vi "te_writeVal.vi"(0 "VISA In":refnum<visa-resource-name>, 5 "Hex Address":string="00", 7 "Command":string="01", 9 "Data":i32, 11 "Error In":errorcluster) -> (4 "VISA Out":refnum<visa-resource-name>, 6 "Response Dec":dbl, 8 "Response":dbl, 15 "error out":errorcluster)   [LabVIEW 2018]
doc: "The Basic Serial Read and Write example performs a Serial Port Read, a Serial Port Write, or a combination of these actions. The user selects the actions (read or write) on the front panel. If both are selected, the VI will write the data first, read data, and then close the VISA session that is opened to the port. This VI will wait until the specified number of bytes is received at the port. Only the number of bytes specified will be read.\n\nINSTRUCTIONS:\n1) Select the serial resource and configuration parameters (baud rate, data bits, parity, stop bits, flow control).\n2) Select the operations to be performed. \n3) Connect the serial port to your device. If no device is available, perform a loopback test by doing one of the following. Short pins 2 and 3 on a RS-232 cable or short pin 4 to pin 8 and pin 5 to pin 9 on a RS-485/422 cable. \n4) Run the VI to see the data read. (The \"read string\" will match the \"string to write\" if a loopback test was performed.)\n\nNote: The parameters set for the serial port must match the parameters of the connected instrument or device. In this example, the bytes to read parameter specifies the number of bytes that the serial port reads. If there were more bytes at the port than the number specified in bytes to read, those bytes would not be read. Also, if you specify to read more bytes than the number of bytes actually read, you might receive a timeout error message.\n\nOn the block diagram, the Configure Serial Port VI sets the configuration parameters. The front panel displays the controls used to configure the basic parameters, such as baud rate, data bits, and parity. Constants configure the other parameters the user probably does not need set. After the VISA Configure Serial Port VI opens the VISA session and configures the port, the VI passes the VISA resource name to other VIs that perform operations on that VISA resource. The VISA Write function sends a command to the serial device and the VISA Read function returns data based on the command. The VISA Close function then closes the reference to the serial device. It is important to close the reference; otherwise communication through with that port through protocols other than VISA might not be possible."
panel:
  out "Response Hex":string
  out "Checksum":string
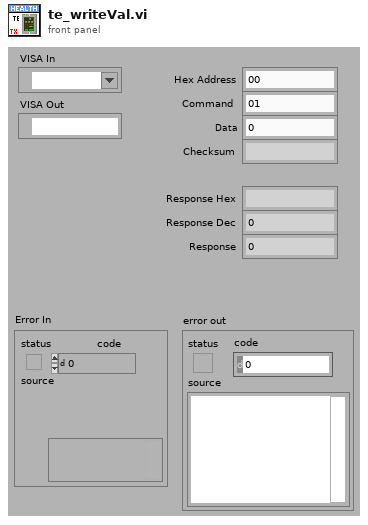
[diagram p1: front panel]
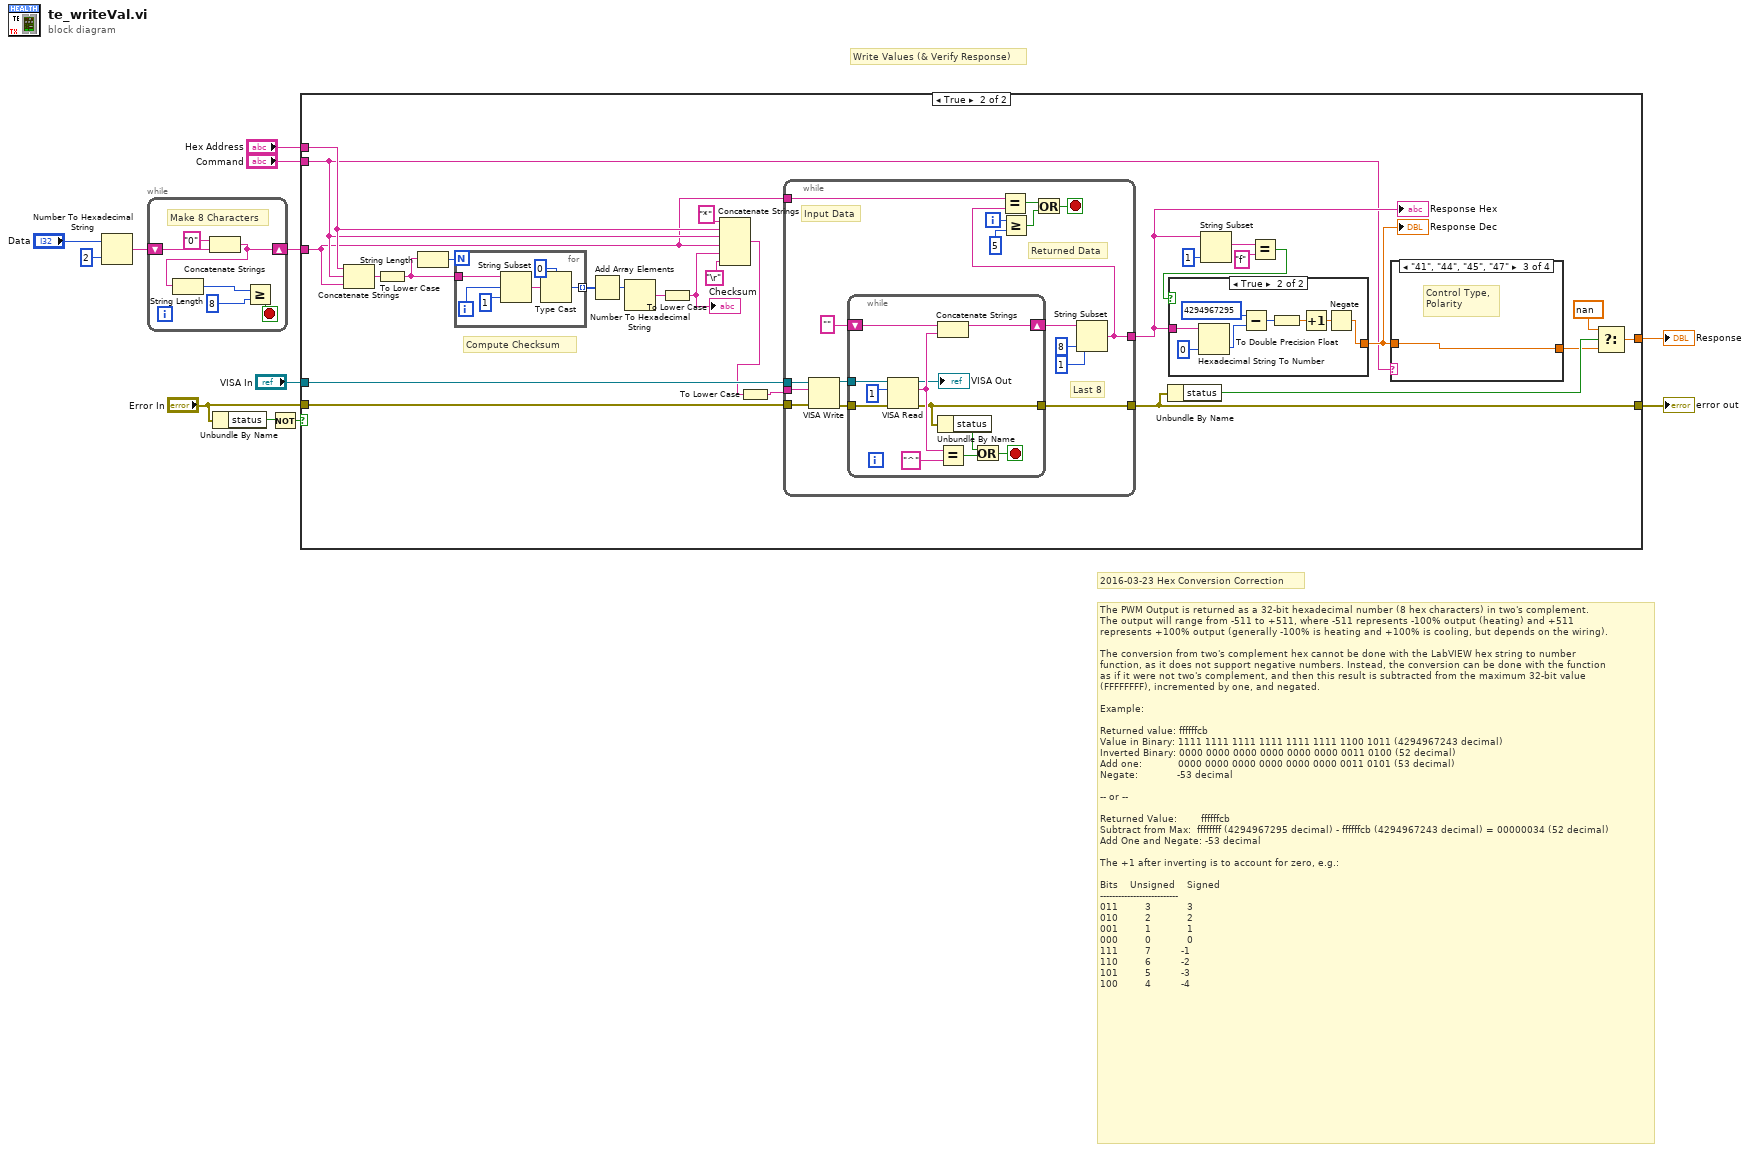
[diagram p0: block diagram]
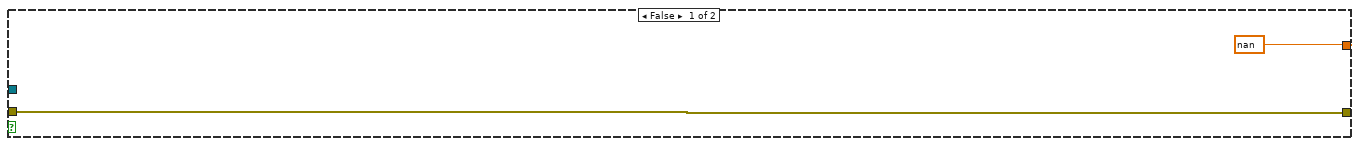
[diagram p2: hidden frame]
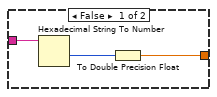
[diagram p3: hidden frame]
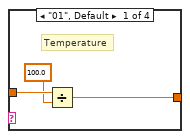
[diagram p4: hidden frame]
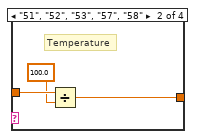
[diagram p5: hidden frame]
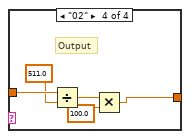
[diagram p6: hidden frame]
diagram:
  # "Write Values (& Verify Response)"
  # "2016-03-23 Hex Conversion Correction"
  # "The PWM Output is returned as a 32-bit hexadecimal number (8 hex characters) in two's complement.\nThe output will range from -511 to +511, where -511 represents -100% output (heating) and +511\nrepresents +100% output (generally -100% is heating and +100% is cooling, but depends on the wiring).\n\nThe conversion from two's complement hex cannot be done with the LabVIEW hex string to number\nfunction, as it does not support negative numbers. Instead, the conversion can be done with the function\nas if it were not two's complement, and then this result is subtracted from the maximum 32-bit value\n(FFFFFFFF), incremented by one, and negated.\n\nExample:\n\nReturned value: ffffffcb\nValue in Binary: 1111 1111 1111 1111 1111 1111 1100 1011 (4294967243 decimal)\nInverted Binary: 0000 0000 0000 0000 0000 0000 0011 0100 (52 decimal)\nAdd one:            0000 0000 0000 0000 0000 0000 0011 0101 (53 decimal)\nNegate:             -53 decimal\n\n-- or --\n\nReturned Value:        ffffffcb\nSubtract from Max:  ffffffff (4294967295 decimal) - ffffffcb (4294967243 decimal) = 00000034 (52 decimal)\nAdd One and Negate: -53 decimal                \n\nThe +1 after inverting is to account for zero, e.g.:\n\nBits    Unsigned    Signed\n--------------------------\n011         3            3\n010         2            2\n001         1            1\n000         0            0\n111         7          -1\n110         6          -2\n101         5          -3\n100         4          -4"
  n1 = Number To Hexadecimal String(1:i16 2 ("width (-)"), 2:"Data") -> (0:w3:string)
  n2 = while {
    shift-right: [w16] -> w9
    shift-left: w3 -> [w18]
    stop <- w13 stop-if-true
    # "Make 8 Characters"
    n3 = Concatenate Strings("0" ("string"), w18) -> (w16:string)
    n4 = String Length(string=w16) -> (length=w14:i32)
    n5 = Greater Or Equal?(x=w14, y=8) -> (x >= y?=w13:bool)
  }
  n6 = Unbundle By Name("Error In") -> ("status"=w11:bool)
  n7 = Not(x=w11) -> (.not. x?=w12:bool)
  n8 = case shown="True" w12 {
    tunnel: "VISA In" -> [_ w46]
    tunnel: "Error In" -> [w20 w45]
    tunnel: [w20 w43] -> w10
    tunnel: w9 -> [_ w27]
    tunnel: [nan ("t") w30] -> w8
    tunnel: "Hex Address" -> [_ w29]
    tunnel: "Command" -> [_ w28]
    frame False {
    }
    frame True {
      # "Compute Checksum"
      n9 = Concatenate Strings(w29, w28, w27) -> (w35:string)
      n10 = To Lower Case(string=w35) -> (all lower case string=w37:string)
      n11 = String Length(string=w37) -> (length=w40:i32)
      n12 = for {
        N: w40 -> [_]
        tunnel: w37 -> [w104]
        tunnel: [w100] -> w39 mode=indexing
        i -> [w103]
        n13 = String Subset(string=w104, offset (0)=w103, length (rest)=1 ("length (rest)")) -> (substring=w101:string)
        n14 = Type Cast(type=u8 0, x=w101) -> (*(type *) &x=w100:u8)
      }
      n15 = Add Array Elements(numeric array=w39) -> (sum=w38:u8)
      n16 = Number To Hexadecimal String(2:w38) -> (0:w36:string)  [unwired: 1 in]
      n17 = To Lower Case(string=w36) -> (all lower case string=w34:string)
      "Checksum" <- w34
      n18 = Concatenate Strings("*", w29, w28, w27, w34, "\r") -> (w21:string)
      n19 = To Lower Case(string=w21) -> (all lower case string=w22:string)
      n20 = while {
        tunnel: w22 -> [w64]
        tunnel: w46 -> [w63]
        tunnel: w45 -> [w62]
        tunnel: [w61] -> w43
        tunnel: [w48] -> w32
        tunnel: w27 -> [w60]
        i -> [w49]
        stop <- w50 stop-if-true
        # "Last 8"
        # "Returned Data"
        # "Input Data"
        n21 = VISA Write(VISA resource name=w63, write buffer=w64, error in (no error)=w62) -> (VISA resource name out=w59:refnum<visa-resource-name>, error out=w58:errorcluster)  [unwired: 1 out]
        n22 = while {
          tunnel: [w67] -> w61
          tunnel: w59 -> [w69]
          tunnel: w58 -> [w75]
          shift-right: [w73] -> w54
          shift-left: "" ("read buffer") -> [w74]
          stop <- w70 stop-if-true
          n23 = VISA Read(VISA resource name=w69, byte count=u32 1, error in (no error)=w75) -> (VISA resource name out=→"VISA Out":refnum<visa-resource-name>, read buffer=w72:string, error out=w67:errorcluster)  [unwired: 1 out]
          n24 = Concatenate Strings(w74, w72) -> (w73:string)
          n25 = Unbundle By Name(w67) -> ("status"=w68:bool)
          n26 = Equal?(x=w72, y="^") -> (x = y?=w66:bool)
          n27 = Or(x=w68, y=w66) -> (x .or. y?=w70:bool)
        }
        n28 = Greater Or Equal?(x=w49, y=5) -> (x >= y?=w52:bool)
        n29 = String Subset(string=w54, offset (0)=1, length (rest)=8 ("length (rest)")) -> (substring=w48:string)
        n30 = Equal?(x=w60, y=w48) -> (x = y?=w51:bool)
        n31 = Or(x=w51, y=w52) -> (x .or. y?=w50:bool)
      }
      "Response Hex" <- w32
      n32 = Unbundle By Name(w43) -> ("status"=w44:bool)
      n33 = String Subset(string=w32, length (rest)=1 ("length (rest)")) -> (substring=w24:string)  [unwired: 1 in]
      n34 = Equal?(x=w24, y="f") -> (x = y?=w26:bool)
      n35 = case shown="True" w26 {
        tunnel: [w78 w82] -> w31
        tunnel: w32 -> [w79 w86]
        frame False {
          n36 = Hexadecimal String To Number(string=w79) -> (number=w77:u32)  [unwired: 2 in, 1 out]
          n37 = To Double Precision Float(number=w77) -> (double precision float=w78:dbl)
        }
        frame True {
          n38 = Hexadecimal String To Number(string=w86, default (0uL)=u32 0 ("default (0 U32)")) -> (number=w84:u32)  [unwired: 1 in, 1 out]
          n39 = Subtract(x=u32 4294967295, y=w84) -> (x-y=w83:u32)
          n40 = To Double Precision Float(number=w83) -> (double precision float=w81:dbl)
          n41 = Increment(x=w81) -> (x+1=w80:dbl)
          n42 = Negate(x=w80) -> (-x=w82:dbl)
        }
      }
      "Response Dec" <- w31
      n43 = case shown="\"41\", \"44\", \"45\", \"47\"" w28 {
        tunnel: w31 -> [w90 w93 w94 w99]
        tunnel: [w88 w91 w94 w95] -> w33
        frame "01", Default {
          # "Temperature"
          n44 = Divide(x=w90, y=100.0) -> (x/y=w88:dbl)
        }
        frame "51", "52", "53", "57", "58" {
          # "Temperature"
          n45 = Divide(x=w93, y=100.0) -> (x/y=w91:dbl)
        }
        frame "41", "44", "45", "47" {
          # "Control Type,\nPolarity"
        }
        frame "02" {
          # "Output"
          n46 = Divide(x=w99, y=511.0) -> (x/y=w97:dbl)
          n47 = Multiply(x=w97, y=100.0) -> (x*y=w95:dbl)
        }
      }
      n48 = Select(t=nan, s=w44, f=w33) -> (s? t:f=w30:dbl)
    }
  }
  "error out" <- w10
  "Response" <- w8
